vi "Do Action.vi"(4 "error in (no error)":errorcluster, 6 "Array in":refnum<class>[](array[class]), 7 "Act_Get One in":refnum<class "Act_Get One.lvclass">) -> (0 "error out":errorcluster, 2 "Array out":refnum<class>[](array[class]), 3 "Act_Get One out":refnum<class "Act_Get One.lvclass">)   [LabVIEW 2014, in "Act_Get One.lvclass"]
uses:
  Act_Get One.lvclass
  Act_Get One.lvclass/Act_Get One.ctl
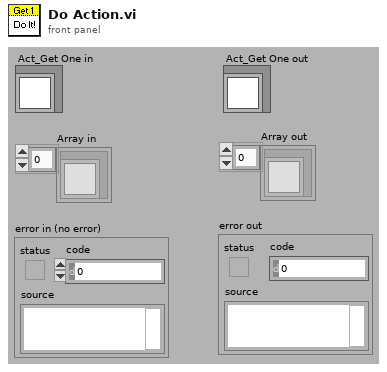
[diagram p1: front panel]
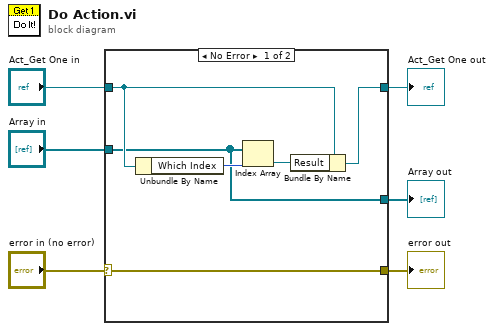
[diagram p0: block diagram]
diagram:
  n1 = case shown="No Error" "error in (no error)" {
    selector: "error in (no error)" -> [w7 w15]
    tunnel: "Array in" -> [w8 w14]
    tunnel: "Act_Get One in" -> [w11 w13]
    tunnel: [w9 w13] -> w3
    tunnel: [w8 w14] -> w2
    tunnel: [w7 w15] -> w1
    frame No Error {
      n2 = Unbundle By Name(w11) -> ("Which Index"=w12:i32)
      n3 = Index Array(array=w8, index=w12) -> (element=w10:refnum<class>)
      n4 = Bundle By Name(cluster=w11, "Result"=w10) -> (w9:refnum<class "Act_Get One.lvclass">)
    }
    frame Error {
    }
  }
  "error out" <- w1
  "Array out" <- w2
  "Act_Get One out" <- w3
